vi "Finish.vi"   [LabVIEW 2014]
doc: "This VI is called just before exiting. It is expected to close I/O refnum, save collected data, etc."
uses:
  <vilib>/Platform/NI_3dgraph.lvlib
  <vilib>/Utility/file.llb/Write To Spreadsheet File (DBL).vi
types:
  T1 = typedef "WPI_JoystickDevRef.ctl" = cluster{"Device":T2}
  T2 = typedef "WPI_JoystickDeviceEnum.ctl" = enum16{"USB 0", "USB 1", "USB 2", "USB 3", "USB 4", "USB 5"}
  T3 = typedef "WPI_RobotDriveDevRef.ctl" = cluster{"DevStatus":errorcluster, "Motors[]":T4[], "Square Inputs":bool, "Max Output":dbl}
  T4 = typedef "WPI_MotorControlDeviceRef.ctl" = cluster{"DeviceStatus":errorcluster, "Type":T5, "PWM":cluster{"Controller":T6, "PWM Channel":T7, "DeadBand":T8}, "CAN":cluster{"Device Number":u8, "Control Mode":T9, "Semaphore":T10, "Max Vout":dbl, "TalonSRX Control Mode":T11}, "Invert":bool, "TransformRef":T12, "InvTransformRef":T12}
  T5 = typedef "WPI_MotorControlType.ctl" = enum16{"PWM", "CAN", "CANTalonSRX"}
  T6 = typedef "FPGA_TypedefDigitalModule.ctl" = enum16{"Controller 1"}
  T7 = typedef "FPGA_DIOPWMChannel.ctl" = enum8{"PWM 0", "PWM 1", "PWM 2", "PWM 3", "PWM 4", "PWM 5", "PWM 6", "PWM 7", "PWM 8", "PWM 9", "PWM MXP 0", "PWM MXP 1", "PWM MXP 2", "PWM MXP 3", "PWM MXP 4", "PWM MXP 5", "PWM MXP 6", "PWM MXP 7", "PWM MXP 8", "PWM MXP 9", "Invalid"}
  T8 = typedef "WPI_PWMDeadband.ctl" = cluster{"Name":string, "maxPositivePwm":i32, "minPositivePwm":i32, "centerPwm":i32, "maxNegativePwm":i32, "minNegativePwm":i32, "angularRange":u16}
  T9 = typedef "WPI_CANJaguar_ControlMode.ctl" = enum8{"Percent VBus", "Current", "Speed", "Position", "Voltage"}
  T10 = typedef "Semaphore RefNum" = refnum<k1>
  T11 = typedef "WPI_CANTalonSRX_APIControlMode.ctl" = enum8{"Percent VBus", "Speed", "Position", "Slave", "Unchanged / Invalid"}
  T12 = typedef "WPI_PWMTransform_ConPane.ctl" = refnum<vi>
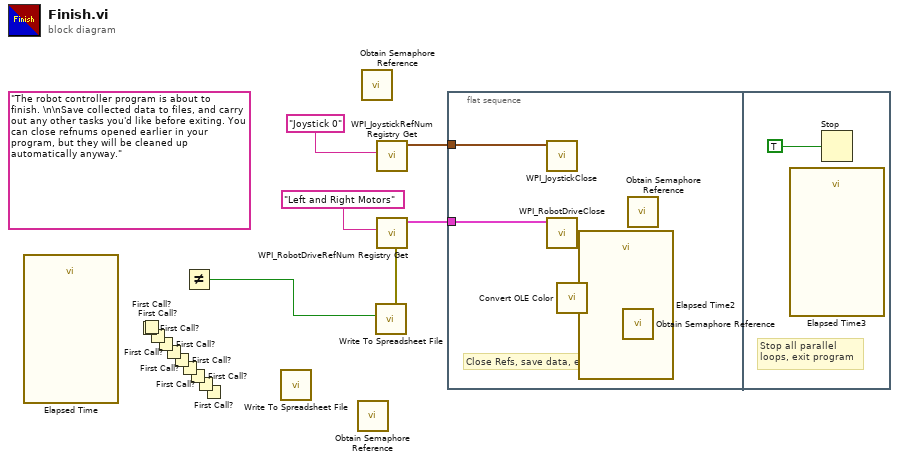
[diagram p0: block diagram]
diagram:
  (unwired) "The robot controller program is about to finish. \n\nSave collected data to files, and carry out any other tasks you'd like before exiting. You can close refnums opened earlier in your program, but they will be cleaned up automatically anyway."
  n1 = call "Elapsed Time"() -> ()  [unwired: 12 in, 8 out]
  n2 = First Call?() -> ()  [unwired: 1 out]
  n3 = First Call?() -> ()  [unwired: 1 out]
  n4 = First Call?() -> ()  [unwired: 1 out]
  n5 = First Call?() -> ()  [unwired: 1 out]
  n6 = First Call?() -> ()  [unwired: 1 out]
  n7 = First Call?() -> ()  [unwired: 1 out]
  n8 = First Call?() -> ()  [unwired: 1 out]
  n9 = First Call?() -> ()  [unwired: 1 out]
  n10 = Not Equal?() -> (x != y?=w2:bool)  [unwired: 2 in]
  n11 = First Call?() -> ()  [unwired: 1 out]
  n12 = First Call?() -> ()  [unwired: 1 out]
  n13 = call-poly <vilib>:"Write To Spreadsheet File.vi"() -> ()  [unwired: 8 in, 1 out]
  n14 = call <vilib>:"Obtain Semaphore Reference.vi"() -> ()  [unwired: 5 in, 3 out]
  n15 = call <vilib>:"Obtain Semaphore Reference.vi"() -> ()  [unwired: 5 in, 3 out]
  n16 = call <vilib>:"WPI_JoystickRefNum Registry Get.vi"("refnum name"="Joystick 0") -> ("JoystickDevRef"=w3:T1)  [unwired: 1 in, 9 out]
  n17 = call <vilib>:"WPI_RobotDriveRefNum Registry Get.vi"("refnum name"="Left and Right Motors") -> ("error out"=w1:errorcluster, "RobotDriveDevRef"=w4:T3)  [unwired: 1 in, 8 out]
  n18 = call-poly <vilib>:"Write To Spreadsheet File.vi"("format (%.3f)"=w1, "2D data"=w2) -> ()  [unwired: 6 in, 1 out]
  n19 = flat-sequence {
    tunnel: w4 -> [w8]
    tunnel: w3 -> [w7]
    frame #0 {
      # "Close Refs, save data, etc."
      n20 = call <vilib>:"WPI_JoystickClose.vi"("JoystickDevRef"=w7) -> ()  [unwired: 11 out]
      n21 = call <vilib>:"WPI_RobotDriveClose.vi"("RobotDriveDevRef"=w8) -> ()  [unwired: 1 in, 10 out]
      n22 = call <vilib>:"Convert OLE Color.vi"() -> ()  [unwired: 1 in, 1 out]
      n23 = call "Elapsed Time2"() -> ()  [unwired: 12 in, 8 out]
      n24 = call <vilib>:"Obtain Semaphore Reference.vi"() -> ()  [unwired: 5 in, 3 out]
      n25 = call <vilib>:"Obtain Semaphore Reference.vi"() -> ()  [unwired: 5 in, 3 out]
    }
    frame #1 {
      # "Stop all parallel\nloops, exit program"
      n26 = call "Elapsed Time3"() -> ()  [unwired: 12 in, 8 out]
      n27 = Stop(stop? (T)=TRUE ("Quit")) -> ()
    }
  }
